vi "Defer Panel Updates.vi"(8 "error in (no error)":errorcluster, 11 "IViewable In":refnum<class "IViewable.lvclass">) -> (0 "error out":errorcluster, 3 "IViewable Out":refnum<class "IViewable.lvclass">)   [LabVIEW 2015, in "IViewable.lvlib" / "IViewable.lvclass"]
uses:
  IViewable.lvclass
  IViewable.lvclass/IViewable.ctl
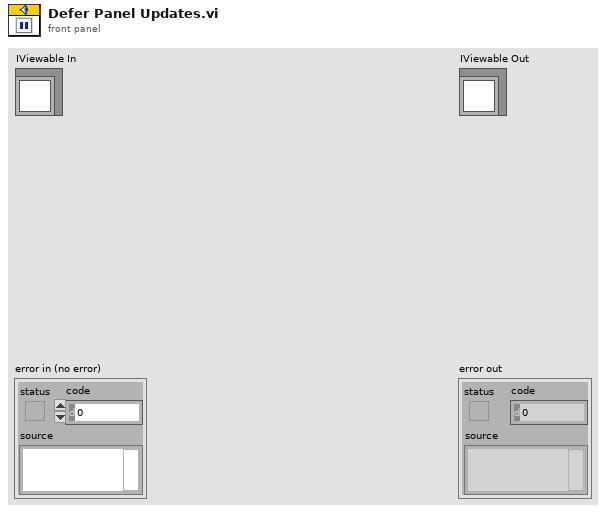
[diagram p1: front panel]
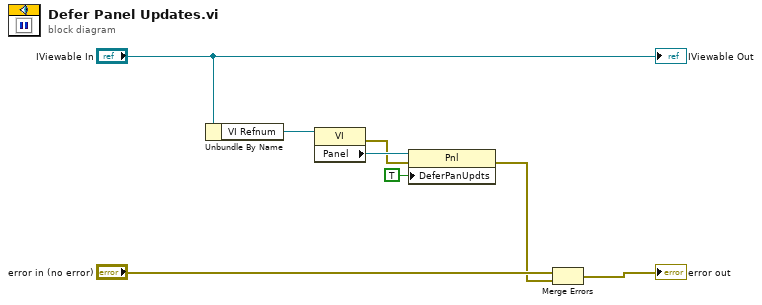
[diagram p0: block diagram]
diagram:
  n1 = Unbundle By Name("IViewable In") -> ("VI Refnum"=w5:refnum<vi>)
  n2 = property class="VI"(reference=w5) -> (error out=w3:errorcluster, "Panel"=w4:refnum<vi>)  [unwired: 1 in, 1 out]
  n3 = property class="Pnl"(reference=w4, error in=w3, "DeferPanUpdts"=TRUE ("Defer Panel Updates")) -> (error out=w2:errorcluster)  [unwired: 1 out]
  n4 = Merge Errors("error in (no error)", w2) -> (→"error out":errorcluster)
  "IViewable Out" <- "IViewable In"
